vi "Draw.vi"(8 "error in (no error)":errorcluster, 10 "picture in (empty picture)":picture, 11 "Geometric Object in":refnum<class "Graphics Object.lvclass">) -> (0 "error out":errorcluster, 2 "picture out":picture, 3 "Geometric Object out":refnum<class "Graphics Object.lvclass">)   [LabVIEW 2018, in "Graphics Object.lvclass"]
doc: "A method for drawing a graphics object"
uses:
  Graphics Object.lvclass
panel:
  # "expressionflow.com"
  # "Copyright (c) 2008 Tomi Maila. All rights reserved."
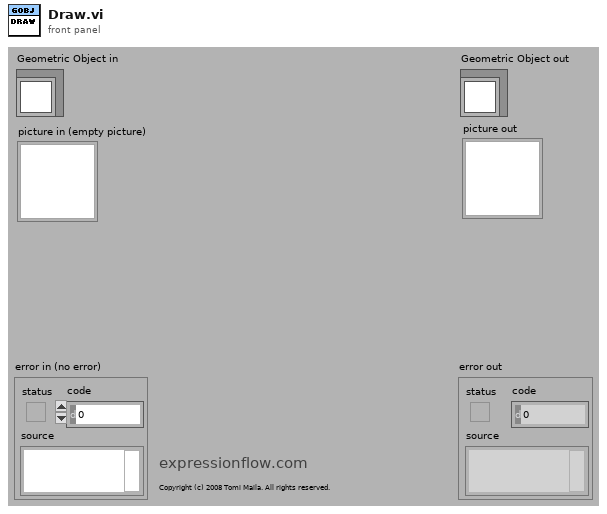
[diagram p1: front panel]
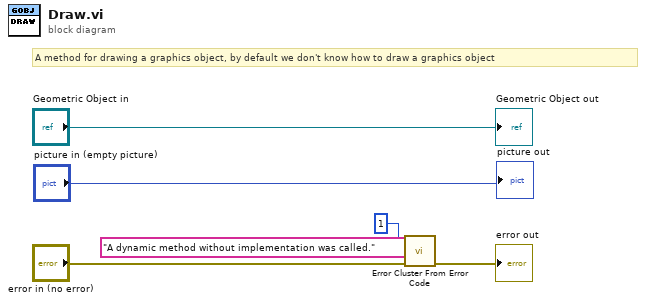
[diagram p0: block diagram]
diagram:
  # "A method for drawing a graphics object, by default we don't know how to draw a graphics object"
  n1 = call <vilib>:"Error Cluster From Error Code.vi"("error in (no error)"="error in (no error)", "error message (\"\")"="A dynamic method without implementation was called." ("error message (\"\")"), "error code (0)"=1) -> ("error out"=→"error out":errorcluster)  [unwired: 6 in]
  "Geometric Object out" <- "Geometric Object in"
  "picture out" <- "picture in (empty picture)"
